vi "Teleop.vi"(8 "error in (no error)":errorcluster, 9 "Joystick Data":T2, 10 "Robot Data In":T1, 11 "Robot in":refnum<class "Robot.lvclass">) -> (0 "error out":errorcluster, 2 "Robot Data Out":T1, 3 "Robot out":refnum<class "Robot.lvclass">)   [LabVIEW 2019, in "Robot.lvlib" / "Robot.lvclass"]
uses:
  Robot.lvclass
  Joysticks/Controls/JoystickData.ctl
  TypeDefs/RobotObjects.ctl
  Drive/Tank Drive/Tank Drive.lvclass
  Pnematics control/Pneumatics.lvclass
  Vision/Vision.lvclass
  Joysticks/Joysticks.lvclass
  Elevator/Elevator.lvclass
  Hatch/Hatch.lvclass
  Cargo/Cargo.lvclass
  DriveOld/Drive.lvclass
  Control Panel/Control Panel.lvclass
  Climber/Climber.lvclass
  Turret/Turret.lvclass
  PowerCellHandler/Power Cell Handler.lvclass
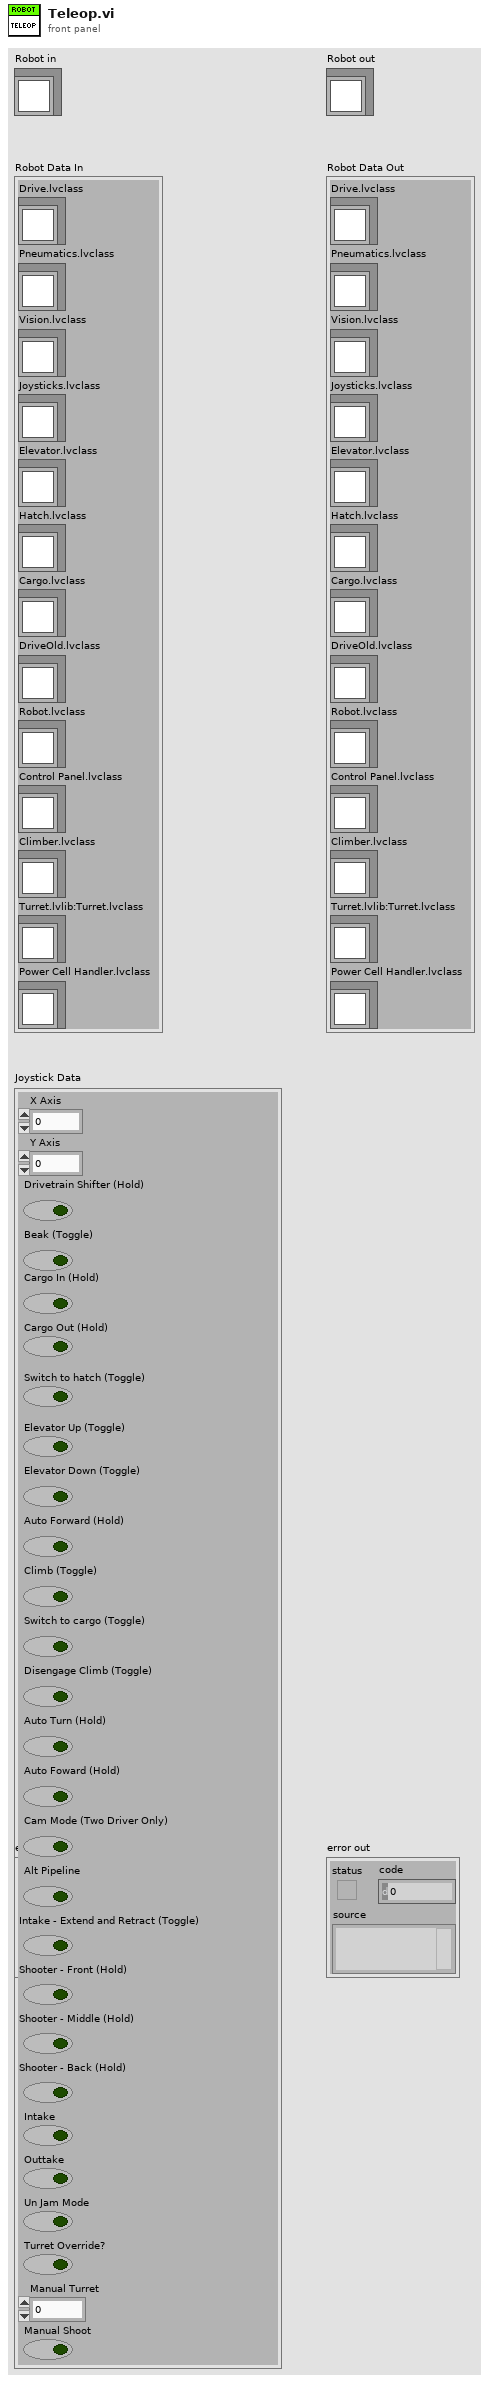
[diagram p1: front panel]
types:
  T1 = typedef "RobotObjects.ctl" = cluster{"Drive.lvclass":refnum<class "Tank Drive.lvclass">, "Pneumatics.lvclass":refnum<class "Pneumatics.lvclass">, "Vision.lvclass":refnum<class "Vision.lvclass">, "Joysticks.lvclass":refnum<class "Joysticks.lvclass">, "Elevator.lvclass":refnum<class "Elevator.lvclass">, "Hatch.lvclass":refnum<class "Hatch.lvclass">, "Cargo.lvclass":refnum<class "Cargo.lvclass">, "DriveOld.lvclass":refnum<class "Drive.lvclass">, "Robot.lvclass":refnum<class "Robot.lvclass">, "Control Panel.lvclass":refnum<class "Control Panel.lvclass">, "Climber.lvclass":refnum<class "Climber.lvclass">, "Turret.lvlib:Turret.lvclass":refnum<class "Turret.lvclass">, "Power Cell Handler.lvclass":refnum<class "Power Cell Handler.lvclass">}
  T2 = typedef "Joysticks.lvlib/Joysticks.lvclass/JoystickData.ctl" = cluster{"X Axis ":dbl, "Y Axis":dbl, "Drivetrain Shifter (Hold)":bool, "Beak (Toggle)":bool, "Cargo In (Hold)":bool, "Cargo Out (Hold)":bool, "Switch to hatch (Toggle)":bool, "Elevator Up (Toggle)":bool, "Elevator Down (Toggle)":bool, "Auto Forward (Hold)":bool, "Climb (Toggle)":bool, "Switch to cargo (Toggle)":bool, "Disengage Climb (Toggle)":bool, "Auto Turn (Hold)":bool, "Auto Foward (Hold)":bool, "Cam Mode (Two Driver Only)":bool, "Alt Pipeline":bool, "Intake - Extend and Retract (Toggle)":bool, "Shooter - Front (Hold)":bool, "Shooter - Middle (Hold)":bool, "Shooter - Back (Hold)":bool, "Intake":bool, "Outtake":bool, "Un Jam Mode":bool, "Turret Override?":bool, "Manual Turret":dbl, "Manual Shoot":bool}
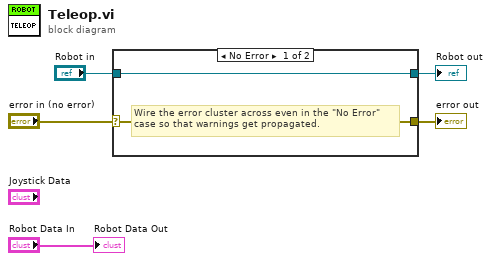
[diagram p0: block diagram]
diagram:
  n1 = case shown="No Error" "error in (no error)" {
    selector: "error in (no error)" -> [w6 w9]
    tunnel: [w6 w9] -> w4
    tunnel: [w7 w8] -> w2
    tunnel: "Robot in" -> [w7 w8]
    frame No Error {
      # "Wire the error cluster across even in the \"No Error\"\ncase so that warnings get propagated."
    }
    frame Error {
    }
  }
  "error out" <- w4
  "Robot out" <- w2
  "Robot Data Out" <- "Robot Data In"
